vi "rqcBob Alice Delay Line Test (Low Level Example).vi"() -> ()   [LabVIEW 2018]
uses:
  FPGA/rqcBob/Custom Controls/Pulse Train/rqcBob Pulse Train Config.ctl
  FPGA/rqcBob/Custom Controls/Pulse Train/rqcBob Pulse Train.Generation Mode.ctl
  FPGA/rqcBob/Custom Controls/Pulse Train/rqcBob Pulse Train.First Pulse Delay Mode.ctl
  FPGA/rqcBob/Custom Controls/rqcBob Window Config.ctl
  Shared/Shared FPGA Lib/Shared Logic/Custom Controls/rqc Random Generator.parameters.ctl
  Shared/Shared FPGA Lib/Shared Logic/Custom Controls/rqc Random Generator.value type.ctl
  FPGA/rqcBob/Custom Controls/rqcBob Modulator Config.ctl
  Custom Controls/rqcBob States.ctl
  FPGA/rqcBob/Custom Controls/rqcBob Trigger Type.ctl
  Shared/Shared Host Lib/rqc ServiceNET/Custom Controls/rqc ServiceNET command.ctl
  Shared/Shared Host Lib/rqc ServiceNET/Bob/Custom Controls/rqcBob ServiceNET control.ctl
  <vilib>/FPGAPlugInAG/PCIe-7820R/niLvFpga_Open_PCIe-7820R.vi
  <vilib>/rvi/interface/common/dynamic/niFpgaDynamicAddResources.vi
  Low Level API/Configuration/Photon Detector/Detection FIFOs config/rqcBob Configure PD Detect FIFO (1PD PD1).vi
  Low Level API/Read/Read PD Detection FIFO/rqcBob Read PD Detection FIFO (1PD PD1).vi
  Shared/Shared Host Lib/rqc ServiceNET/Bob/rqcBob Send Data/rqcBob ServiceNET Send Data U32.vi
  <vilib>/FPGAPlugInAG/Dynamic/niLvFpga_Close_Dynamic.vi
  <vilib>/rvi/interface/nirviOpenFPGA/nirviOpenFPGA.xnode
  FPGA Bitfiles/rqcBob (FPGA) 7820 v 4.0.0.lvbitx
  <vilib>/rvi/interface/nirviCloseFPGA/nirviCloseFPGA.xnode
panel:
  in  "modulator.clock delay":fxp<+,4,4>
  out "current States":T1=enum."App.Stop"
  out "error out":errorcluster
  out "Connected to Alice":bool
  in  "Stop":bool
  in  "modulator.config":T2={"modulator.start"=1000, "modulator.stop"=3700}
  in  "PD.detection window":u8=25
  in  "rndGen.parameters":T3={"value type"=enum."constant", "constant"=0, "num of levels"=0, "levels values"=[0, 0, 0, 0]}
  in  "window.config":T5={"window.open"=2530, "window.close"=2531}
  in  "train.configuration":T6={"period"=4000, "num of pulses"=3, "mode"=enum."train sequence.single", "num of trains"=1000, "first pulse delay mode"=enum."every train", "first pulse delay"=55}
  in  "Port:":u16=5020
  in  "Alice's IP address":string="192.168.0.175"
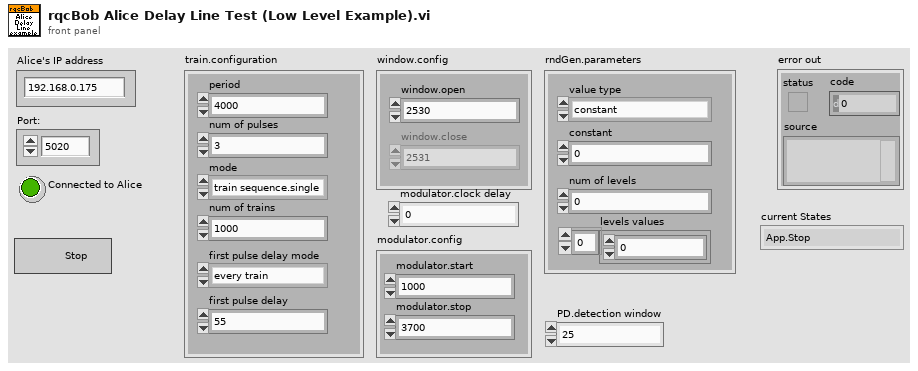
[diagram p1: front panel]
types:
  T1 = typedef "rqcBob States.ctl" = enum16{"HW.configure", "HW.sendTrigger", "HW.initiate", "HW.measure", "HW.stop", "NET.create", "NET.connect", "NET.sendCommand", "NET.readCommand", "NET.readData", "NET.close", "App.HandleEvent", "App.HandleError", "App.Stop"}
  T2 = typedef "rqcBob Modulator Config.ctl" = cluster{"modulator.start":u16, "modulator.stop":u16}
  T3 = typedef "rqc Random Generator.parameters.ctl" = cluster{"value type":T4, "constant":u16, "num of levels":u16, "levels values":u16[]}
  T4 = typedef "rqc Random Generator.value type.ctl" = enum16{"random value", "constant"}
  T5 = typedef "rqcBob Window Config.ctl" = cluster{"window.open":u16, "window.close":u16}
  T6 = typedef "rqcBob Pulse Train Config.ctl" = cluster{"period":u16, "num of pulses":u16, "mode":T7, "num of trains":u16, "first pulse delay mode":T8, "first pulse delay":u16}
  T7 = typedef "rqcBob Pulse Train.Generation Mode.ctl" = enum8{"single train", "train sequence.single", "train sequence.wait for trigger", "continuous"}
  T8 = typedef "rqcBob Pulse Train.First Pulse Delay Mode.ctl" = enum8{"none", "every train", "first train"}
  T9 = typedef "rqcBob Trigger Type.ctl" = enum16{"software", "immediate", "DIO"}
  T10 = typedef "rqc ServiceNET command.ctl" = enum8{"NONE", "READY", "START", "PING"}
  T11 = typedef "rqcBob ServiceNET control.ctl" = cluster{"connection ID":refnum<k5>, "connected?":bool, "Alice's IP address":string, "port":u16}
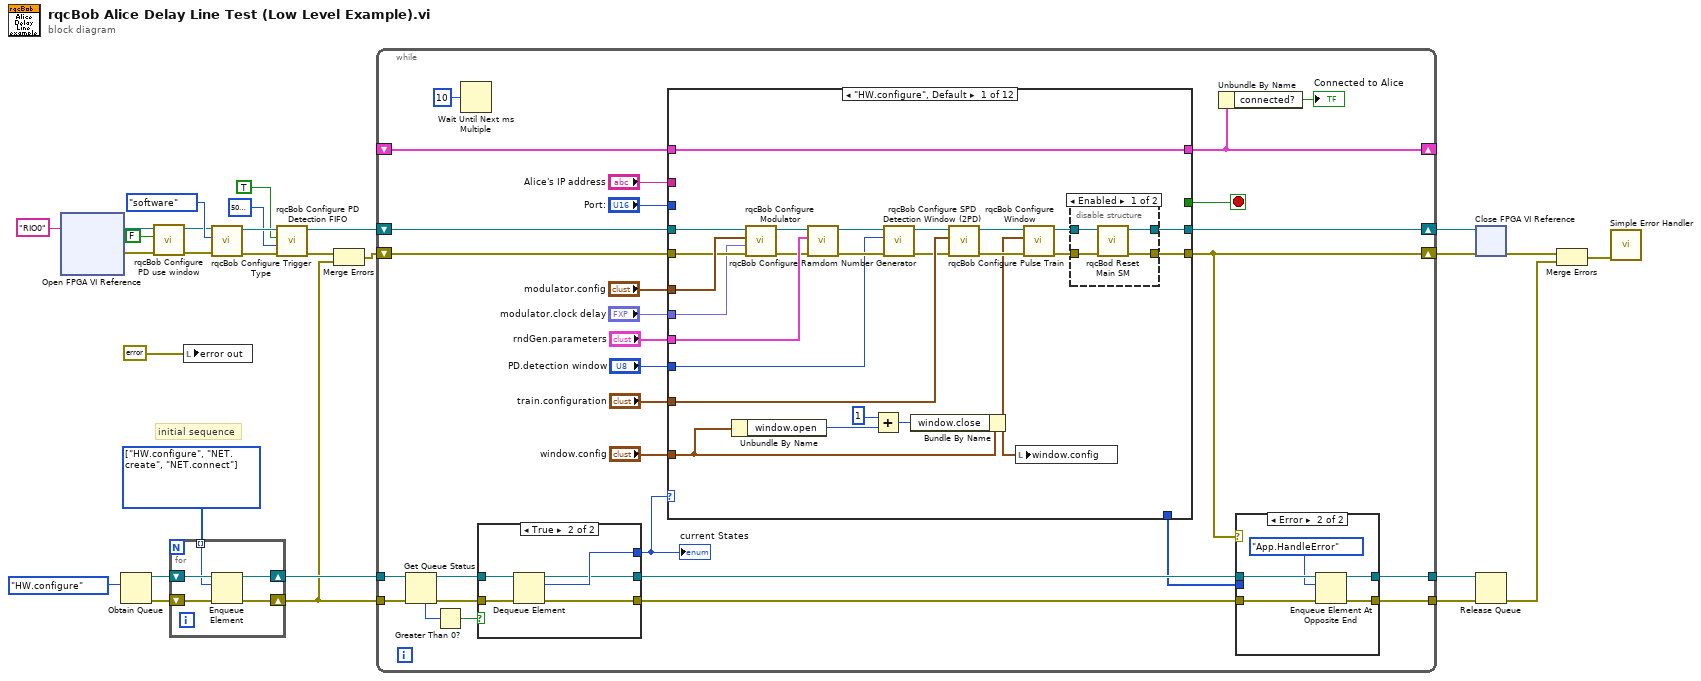
[diagram p0: block diagram]
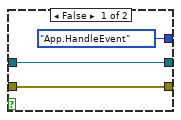
[diagram p2: hidden frame]
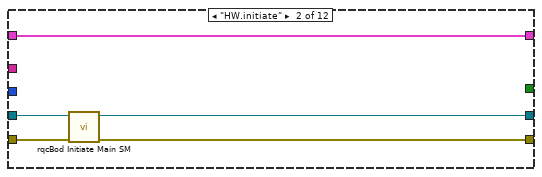
[diagram p4: hidden frame]
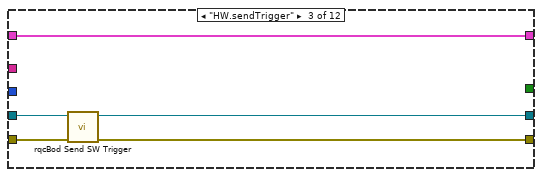
[diagram p5: hidden frame]
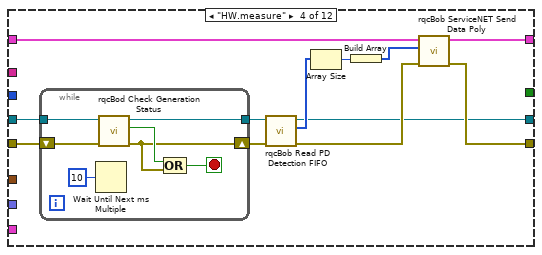
[diagram p6: hidden frame]
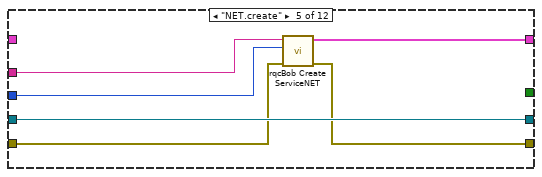
[diagram p7: hidden frame]
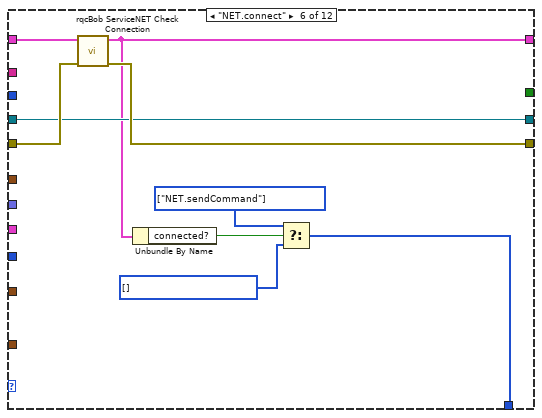
[diagram p8: hidden frame]
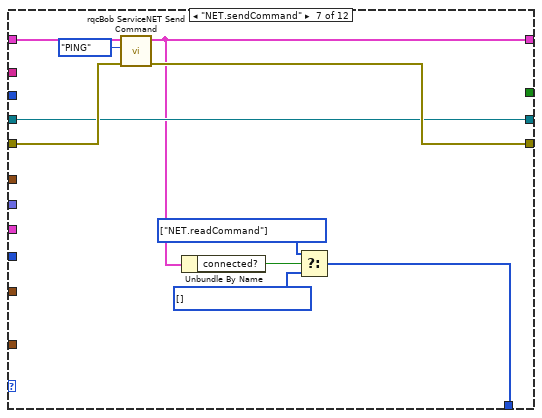
[diagram p9: hidden frame]
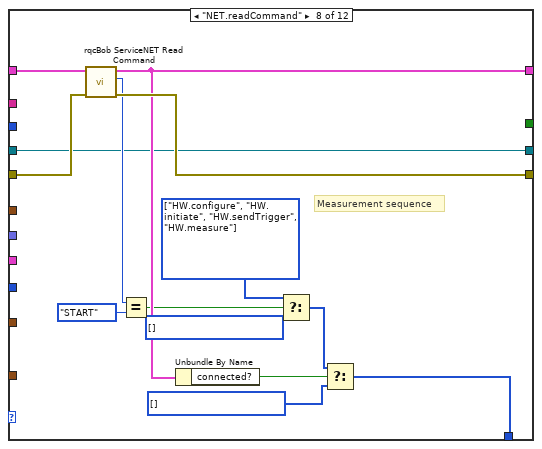
[diagram p10: hidden frame]
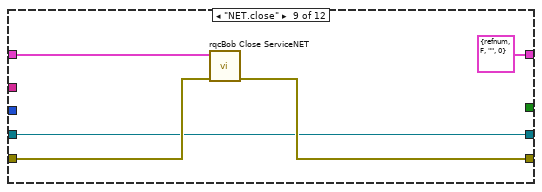
[diagram p11: hidden frame]
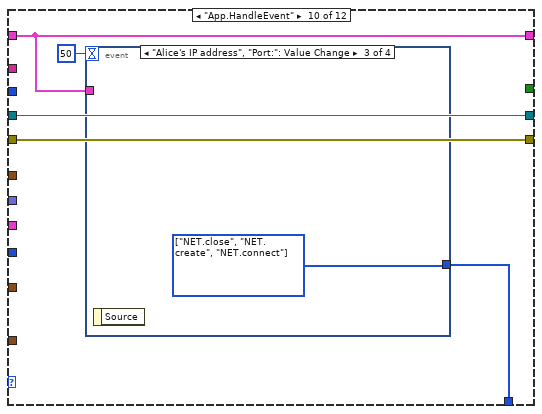
[diagram p12: hidden frame]
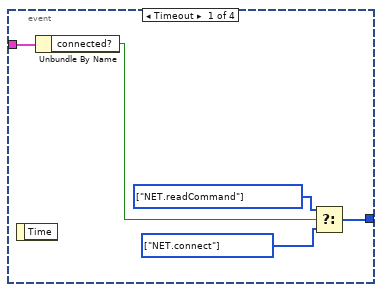
[diagram p13: hidden frame]
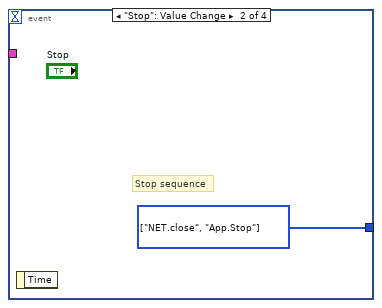
[diagram p14: hidden frame]
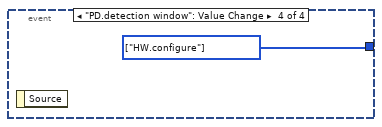
[diagram p15: hidden frame]
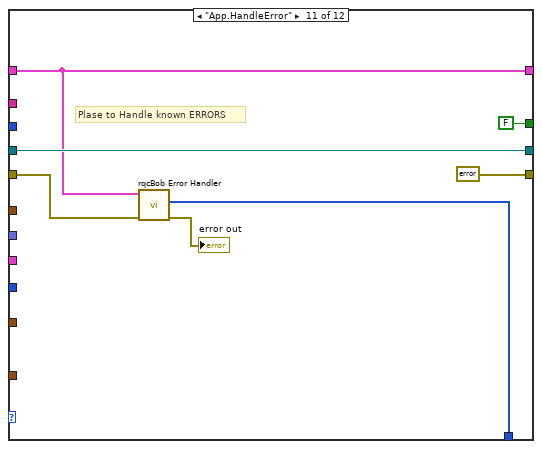
[diagram p16: hidden frame]
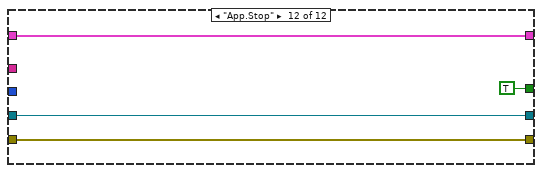
[diagram p17: hidden frame]
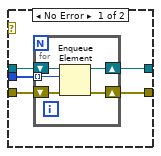
[diagram p18: hidden frame]
diagram:
  w19 = T1[] [enum."HW.configure", enum."NET.create", enum."NET.connect"] items=["HW.configure", "HW.sendTrigger", "HW.initiate", "HW.measure", "HW.stop", "NET.create", "NET.connect", "NET.sendCommand", "NET.readCommand", "NET.readData", "NET.close", "App.HandleEvent", "App.HandleError", "App.Stop"]
  # "initial sequence"
  n1 = xnode "Open FPGA VI Reference"("resource name"="RIO0") -> ("FPGA VI Reference Out"=w9:refnum<k20>, "error out"=w8:errorcluster)  [unwired: 1 in]
  n2 = Obtain Queue(element data type=rqcBob_States."HW.configure" ("rqcBob States")) -> (queue out=w24:refnum<queue>, error out=w23:errorcluster)  [unwired: 4 in, 1 out]
  n3 = call "rqcBob Configure PD use window.vi"("error in"=w8, "PD.use window"=FALSE ("SPD.use detector window"), "FPGA reference in"=w9) -> ("error out"=w25:errorcluster, "FPGA reference out"=w26:refnum<k20>)  [unwired: 7 in]
  n4 = for {
    tunnel: w19 -> [w29] mode=indexing
    shift-right: [w30] -> w21
    shift-left: w24 -> [w33]
    shift-right: [w31] -> w18
    shift-left: w23 -> [w32]
    n5 = Enqueue Element(queue=w33, element=w29, error in (no error)=w32) -> (queue out=w30:refnum<queue>, error out=w31:errorcluster)  [unwired: 1 in, 1 out]
  }
  n6 = local write "error out"(errorcluster {"status"=FALSE, "code"=0, "source"=""} ("error constant")) -> ()
  n7 = call "rqcBob Configure Trigger Type.vi"("error in"=w25, "rqcBob Trigger Type"=rqcBob_Trigger_Type."software", "FPGA reference in"=w26) -> ("error out"=w3:errorcluster, "FPGA reference out"=w5:refnum<k20>)  [unwired: 7 in]
  n8 = call-poly "rqcBob Configure PD Detection FIFO.vi"("error in"=w3, "PD.detect fifo depth"=u32 5000000 ("SPD.detect fifo depth"), "PD.detect fifo write enable"=TRUE ("SPD.detect fifo write enable"), "FPGA reference in"=w5) -> ("error out"=w4:errorcluster, "FPGA reference out"=w6:refnum<k20>)  [unwired: 6 in]
  n9 = Merge Errors(w4, w18) -> (w22:errorcluster)
  n10 = while {
    shift-right: [w43] -> w17
    shift-left: w22 -> [w54]
    shift-right: [w44] -> w16
    shift-left: w6 -> [w41]
    tunnel: w21 -> [w52]
    tunnel: w18 -> [w51]
    tunnel: [w46] -> w15
    tunnel: [w45] -> w14
    shift-right: [w37] -> _
    shift-left: _ -> [w38]
    stop <- w42 stop-if-true
    n11 = Get Queue Status(queue=w52, error in (no error)=w51) -> (queue out=w48:refnum<queue>, error out=w47:errorcluster, # elements in queue=w50:i32)  [unwired: 1 in, 5 out]
    n12 = Greater Than 0?(x=w50) -> (x > 0?=w49:bool)
    n13 = Wait Until Next ms Multiple(millisecond multiple=u32 10) -> ()  [unwired: 1 out]
    n14 = case shown="True" w49 {
      tunnel: w48 -> [w63 w70]
      tunnel: w47 -> [w64 w69]
      tunnel: [rqcBob_States."App.HandleEvent" ("rqcBob States") w68] -> w57
      tunnel: [w63 w67] -> w56
      tunnel: [w64 w66] -> w53
      frame False {
      }
      frame True {
        n15 = Dequeue Element(queue=w70, error in (no error)=w69) -> (queue out=w67:refnum<queue>, element=w68:T1, error out=w66:errorcluster)  [unwired: 1 in, 1 out]
      }
    }
    "current States" <- w57
    n16 = case shown="\"HW.configure\", Default" w57 {
      tunnel: "modulator.config" -> [w89 _ _ _ _ _ _ _ _ _ _ _]
      tunnel: "train.configuration" -> [w88 _ _ _ _ _ _ _ _ _ _ _]
      tunnel: "window.config" -> [w87 _ _ _ _ _ _ _ _ _ _ _]
      tunnel: "rndGen.parameters" -> [w86 _ _ _ _ _ _ _ _ _ _ _]
      tunnel: "PD.detection window" -> [w85 _ _ _ _ _ _ _ _ _ _ _]
      tunnel: [w74 w103 w108 w118 w131 w143 w153 w167 w171 w177 errorcluster {"status"=FALSE, "code"=0, "source"=""} ("error constant") w196] -> w43
      tunnel: w54 -> [w84 w105 w110 w122 w132 w144 w154 w168 w172 w177 w191 w196]
      tunnel: [_ _ _ _ _ w137 w146 w163 _ w176 w190 _] -> w55
      tunnel: [w76 w104 w109 w112 w136 w142 w152 w156 w170 w178 w193 w197] -> w44
      tunnel: [_ _ _ _ _ _ _ _ _ _ FALSE TRUE] -> w42
      tunnel: w41 -> [w83 w106 w111 w123 w136 w142 w152 w156 w170 w178 w193 w197]
      tunnel: "Alice's IP address" -> [_ _ _ _ w135 _ _ _ _ _ _ _]
      tunnel: "Port:" -> [_ _ _ _ w134 _ _ _ _ _ _ _]
      tunnel: [w73 w102 w107 w120 w133 w141 w150 w164 T11 {"connection ID"=refnum, "connected?"=FALSE, "Alice's IP address"="", "port"=0} ("rqcBob ServiceNET control") w175 w192 w195] -> w37
      tunnel: w38 -> [w73 w102 w107 w119 _ w145 w155 w169 w174 w175 w192 w195]
      tunnel: "modulator.clock delay" -> [w71 _ _ _ _ _ _ _ _ _ _ _]
      frame "HW.configure", Default {
        n17 = Unbundle By Name(w87) -> ("window.open"=w95:u16)
        n18 = call "rqcBob Configure Modulator.vi"("error in"=w84, "modulator.clock delay"=w71, "modulator.config"=w89, "FPGA reference in"=w83) -> ("error out"=w82:errorcluster, "FPGA reference out"=w81:refnum<k20>)  [unwired: 6 in]
        n19 = call "rqcBob Configure Ramdom Number Generator.vi"("error in"=w82, "rqcBob rndGen.parameters"=w86, "FPGA reference in"=w81) -> ("error out"=w90:errorcluster, "FPGA reference out"=w91:refnum<k20>)  [unwired: 7 in]
        n20 = Add(x=u16 1, y=w95) -> (x+y=w92:u16)
        n21 = call "rqcBob Configure SPD Detection Window (2PD).vi"("error in"=w90, "PD1.detection window"=w85, "FPGA reference in"=w91) -> ("error out"=w79:errorcluster, "FPGA reference out"=w80:refnum<k20>)  [unwired: 7 in]
        n22 = Bundle By Name(cluster=w87, "window.close"=w92) -> (w78:T5)
        n23 = call "rqcBob Configure Pulse Train.vi"("error in"=w79, "train.configuration"=w88, "FPGA reference in"=w80) -> ("error out"=w93:errorcluster, "FPGA reference out"=w94:refnum<k20>)  [unwired: 6 in, 1 out]
        n24 = local write "window.config"(w78) -> ()
        n25 = call "rqcBob Configure Window.vi"("error in"=w93, "window.config"=w78, "FPGA reference in"=w94) -> ("error out"=w75:errorcluster, "FPGA reference out"=w77:refnum<k20>)  [unwired: 7 in]
        n26 = disable-structure shown="Enabled" {
          disable-tunnel: w77 -> [w99 w101]
          disable-tunnel: [w98 w101] -> w76
          disable-tunnel: w75 -> [w97 w100]
          disable-tunnel: [w96 w100] -> w74
          frame Enabled {
            n27 = call "rqcBod Reset Main SM.vi"("error in"=w97, "FPGA reference in"=w99) -> ("error out"=w96:errorcluster, "FPGA reference out"=w98:refnum<k20>)  [unwired: 8 in]
          }
          frame Disabled {
          }
        }
      }
      frame "HW.initiate" {
        n28 = call "rqcBod Initiate Main SM.vi"("error in"=w105, "FPGA reference in"=w106) -> ("error out"=w103:errorcluster, "FPGA reference out"=w104:refnum<k20>)  [unwired: 8 in]
      }
      frame "HW.sendTrigger" {
        n29 = call "rqcBod Send SW Trigger.vi"("error in"=w110, "FPGA reference in"=w111) -> ("error out"=w108:errorcluster, "FPGA reference out"=w109:refnum<k20>)  [unwired: 8 in]
      }
      frame "HW.measure" {
        n30 = while {
          tunnel: w123 -> [w130]
          shift-right: [w124] -> w115
          shift-left: w122 -> [w129]
          tunnel: [w126] -> w116
          stop <- w125 stop-if-true
          n31 = Wait Until Next ms Multiple(millisecond multiple=u32 10) -> ()  [unwired: 1 out]
          n32 = call "rqcBod Check Generation Status.vi"("error in"=w129, "FPGA reference in"=w130) -> ("error out"=w124:errorcluster, "generation.done"=w127:bool, "FPGA reference out"=w126:refnum<k20>)  [unwired: 7 in]
          n33 = Compound Arithmetic op=OR(w127, w124) -> (w125:bool)
        }
        n34 = call-poly "rqcBob Read PD Detection FIFO.vi"("error in"=w115, "FPGA reference in"=w116) -> ("error out"=w114:errorcluster, "Data"=w113:u32[], "FPGA reference out"=w112:refnum<k20>)  [unwired: 6 in, 1 out]
        n35 = Array Size(array=w113) -> (size(s)=w121:i32)
        n36 = Build Array(w121) -> (w117:i32[])
        n37 = call-poly "rqcBob ServiceNET Send Data Poly.vi"("error in"=w114, "Data"=w117, "rqcBob ServiceNET in"=w119) -> ("error out"=w118:errorcluster, "rqcBob ServiceNET out"=w120:T11)  [unwired: 7 in]
      }
      frame "NET.create" {
        n38 = call "rqcBob Create ServiceNET.vi"("error in"=w132, "port"=w134, "Alice's IP address"=w135) -> ("error out"=w131:errorcluster, "rqcBob ServiceNET control"=w133:T11)  [unwired: 7 in]
      }
      frame "NET.connect" {
        w138 = T1[] [] items=["HW.configure", "HW.sendTrigger", "HW.initiate", "HW.measure", "HW.stop", "NET.create", "NET.connect", "NET.sendCommand", "NET.readCommand", "NET.readData", "NET.close", "App.HandleEvent", "App.HandleError", "App.Stop"] ("f")
        w140 = T1[] [enum."NET.sendCommand"] items=["HW.configure", "HW.sendTrigger", "HW.initiate", "HW.measure", "HW.stop", "NET.create", "NET.connect", "NET.sendCommand", "NET.readCommand", "NET.readData", "NET.close", "App.HandleEvent", "App.HandleError", "App.Stop"]
        n39 = call "rqcBob ServiceNET Check Connection.vi"("error in"=w144, "rqcBob ServiceNET in"=w145) -> ("error out"=w143:errorcluster, "rqcBob ServiceNET out"=w141:T11)  [unwired: 8 in]
        n40 = Unbundle By Name(w141) -> ("connected?"=w139:bool)
        n41 = Select(t=w140, s=w139, f=w138) -> (s? t:f=w137:T1[])
      }
      frame "NET.sendCommand" {
        w147 = T1[] [] items=["HW.configure", "HW.sendTrigger", "HW.initiate", "HW.measure", "HW.stop", "NET.create", "NET.connect", "NET.sendCommand", "NET.readCommand", "NET.readData", "NET.close", "App.HandleEvent", "App.HandleError", "App.Stop"] ("f")
        w148 = T1[] [enum."NET.readCommand"] items=["HW.configure", "HW.sendTrigger", "HW.initiate", "HW.measure", "HW.stop", "NET.create", "NET.connect", "NET.sendCommand", "NET.readCommand", "NET.readData", "NET.close", "App.HandleEvent", "App.HandleError", "App.Stop"] ("f")
        n42 = call "rqcBob ServiceNET Send Command.vi"("error in"=w154, "command"=rqc_ServiceNET_command."PING", "rqcBob ServiceNET in"=w155) -> ("error out"=w153:errorcluster, "rqcBob ServiceNET out"=w150:T11)  [unwired: 7 in]
        n43 = Unbundle By Name(w150) -> ("connected?"=w149:bool)
        n44 = Select(t=w148, s=w149, f=w147) -> (s? t:f=w146:T1[])
      }
      frame "NET.readCommand" {
        w158 = T1[] [] items=["HW.configure", "HW.sendTrigger", "HW.initiate", "HW.measure", "HW.stop", "NET.create", "NET.connect", "NET.sendCommand", "NET.readCommand", "NET.readData", "NET.close", "App.HandleEvent", "App.HandleError", "App.Stop"] ("f")
        w165 = T1[] [] items=["HW.configure", "HW.sendTrigger", "HW.initiate", "HW.measure", "HW.stop", "NET.create", "NET.connect", "NET.sendCommand", "NET.readCommand", "NET.readData", "NET.close", "App.HandleEvent", "App.HandleError", "App.Stop"] ("f")
        w159 = T1[] [enum."HW.configure", enum."HW.initiate", enum."HW.sendTrigger", enum."HW.measure"] items=["HW.configure", "HW.sendTrigger", "HW.initiate", "HW.measure", "HW.stop", "NET.create", "NET.connect", "NET.sendCommand", "NET.readCommand", "NET.readData", "NET.close", "App.HandleEvent", "App.HandleError", "App.Stop"] ("f")
        # "Measurement sequence"
        n45 = call "rqcBob ServiceNET Read Command.vi"("error in"=w168, "rqcBob ServiceNET in"=w169) -> ("error out"=w167:errorcluster, "command"=w162:T10, "rqcBob ServiceNET out"=w164:T11)  [unwired: 6 in, 1 out]
        n46 = Equal?(x=w162, y=rqc_ServiceNET_command."START") -> (x = y?=w160:bool)
        n47 = Unbundle By Name(w164) -> ("connected?"=w166:bool)
        n48 = Select(t=w159, s=w160, f=w158) -> (s? t:f=w157:T1[])
        n49 = Select(t=w157, s=w166, f=w165) -> (s? t:f=w163:T1[])
      }
      frame "NET.close" {
        n50 = call "rqcBob Close ServiceNET.vi"("error in"=w172, "rqcBob ServiceNET control"=w174) -> ("error out"=w171:errorcluster)  [unwired: 9 in]
      }
      frame "App.HandleEvent" {
        n51 = event shown="[2] \"Alice's IP address\", \"Port:\": Value Change" {
          selector: _ -> [_ _ _ _]
          dyn-events: _ -> [_ _ _ _]
          timeout: 50 -> [_ _ _ _]
          tunnel: [w183 w185 w186 w187] -> w176
          tunnel: w175 -> [w184 _ _ _]
          event Timeout {
            w180 = T1[] [enum."NET.connect"] items=["HW.configure", "HW.sendTrigger", "HW.initiate", "HW.measure", "HW.stop", "NET.create", "NET.connect", "NET.sendCommand", "NET.readCommand", "NET.readData", "NET.close", "App.HandleEvent", "App.HandleError", "App.Stop"]
            w181 = T1[] [enum."NET.readCommand"] items=["HW.configure", "HW.sendTrigger", "HW.initiate", "HW.measure", "HW.stop", "NET.create", "NET.connect", "NET.sendCommand", "NET.readCommand", "NET.readData", "NET.close", "App.HandleEvent", "App.HandleError", "App.Stop"]
            n52 = event-data() -> ()  [unwired: 1 in, 1 out]
            n53 = Unbundle By Name(w184) -> ("connected?"=w182:bool)
            n54 = Select(t=w181, s=w182, f=w180) -> (s? t:f=w183:T1[])
          }
          event "Stop": Value Change {
            w185 = T1[] [enum."NET.close", enum."App.Stop"] items=["HW.configure", "HW.sendTrigger", "HW.initiate", "HW.measure", "HW.stop", "NET.create", "NET.connect", "NET.sendCommand", "NET.readCommand", "NET.readData", "NET.close", "App.HandleEvent", "App.HandleError", "App.Stop"]
            # "Stop sequence"
            n55 = event-data() -> ()  [unwired: 1 in, 1 out]
          }
          event "Alice's IP address", "Port:": Value Change {
            w186 = T1[] [enum."NET.close", enum."NET.create", enum."NET.connect"] items=["HW.configure", "HW.sendTrigger", "HW.initiate", "HW.measure", "HW.stop", "NET.create", "NET.connect", "NET.sendCommand", "NET.readCommand", "NET.readData", "NET.close", "App.HandleEvent", "App.HandleError", "App.Stop"]
            n56 = event-data() -> ()  [unwired: 1 in, 1 out]
          }
          event "PD.detection window": Value Change {
            w187 = T1[] [enum."HW.configure"] items=["HW.configure", "HW.sendTrigger", "HW.initiate", "HW.measure", "HW.stop", "NET.create", "NET.connect", "NET.sendCommand", "NET.readCommand", "NET.readData", "NET.close", "App.HandleEvent", "App.HandleError", "App.Stop"]
            n57 = event-data() -> ()  [unwired: 1 in, 1 out]
          }
        }
      }
      frame "App.HandleError" {
        # "Plase to Handle known ERRORS"
        n58 = call "rqcBob Error Handler.vi"("error in (no error)"=w191, "rqcBob ServiceNET control"=w192) -> ("error out"=→"error out":errorcluster, "error sequence"=w190:T1[])  [unwired: 8 in]
      }
      frame "App.Stop" {
      }
    }
    n59 = Unbundle By Name(w37) -> ("connected?"=→"Connected to Alice":bool)
    n60 = case shown="Error" w43 {
      tunnel: w56 -> [w203 w213]
      tunnel: w55 -> [w200 _]
      tunnel: w53 -> [w199 w212]
      tunnel: [w202 w210] -> w46
      tunnel: [w201 w209] -> w45
      frame No Error {
        n61 = for {
          tunnel: w200 -> [w207] mode=indexing
          shift-right: [w205] -> w201
          shift-left: w199 -> [w206]
          shift-right: [w204] -> w202
          shift-left: w203 -> [w208]
          n62 = Enqueue Element(queue=w208, element=w207, error in (no error)=w206) -> (queue out=w204:refnum<queue>, error out=w205:errorcluster)  [unwired: 1 in, 1 out]
        }
      }
      frame Error {
        n63 = Enqueue Element At Opposite End(queue=w213, element=rqcBob_States."App.HandleError", error in (no error)=w212) -> (queue out=w210:refnum<queue>, error out=w209:errorcluster)  [unwired: 1 in, 1 out]
      }
    }
  }
  n64 = xnode "Close FPGA VI Reference"("FPGA VI Reference In"=w16, "error in"=w17) -> ("error out"=w13:errorcluster)
  n65 = Release Queue(queue=w15, error in (no error)=w14) -> (error out=w12:errorcluster)  [unwired: 1 in, 2 out]
  n66 = Merge Errors(w13, w12) -> (w11:errorcluster)
  n67 = call <vilib>:"Simple Error Handler.vi"("error in (no error)"=w11) -> ()  [unwired: 4 in, 5 out]
